vi "WinPositioner.vi"(0 "Display?":bool, 4 "Yoffset 2":dbl, 6 "Xoffset":dbl, 7 "Image":T1, 8 "Y position":dbl(slide) scale=0.0..10.0, 9 "Fine Y position":dbl(slide) scale=0.0..10.0, 10 "Fine X position":dbl(slide) scale=0.0..10.0, 11 "X position":dbl(slide) scale=0.0..10.0) -> (1 "Y position":dbl, 2 "X position":dbl, 5 "CGH_x":T1(plugin-control))   [LabVIEW 2011]
uses:
  <vilib>/vision/Image Controls.llb/IMAQ Image.ctl
panel:
  # "1"
  # "2"
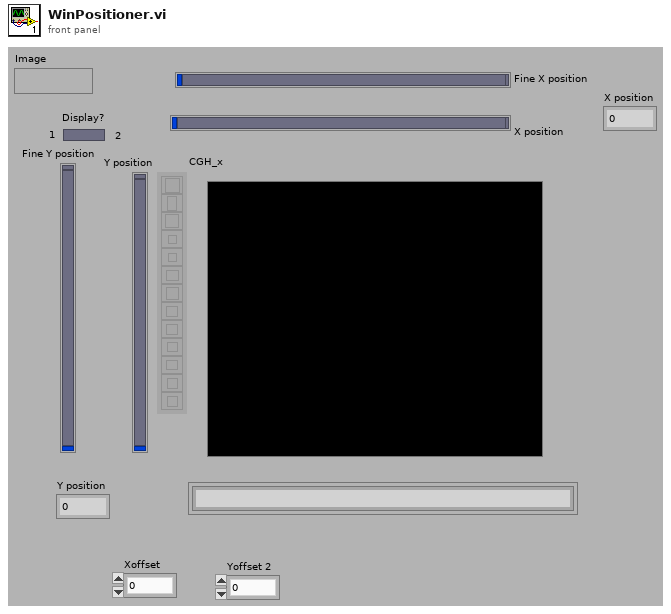
[diagram p1: front panel]
types:
  T1 = typedef "IMAQ Image.ctl" = refnum<image>
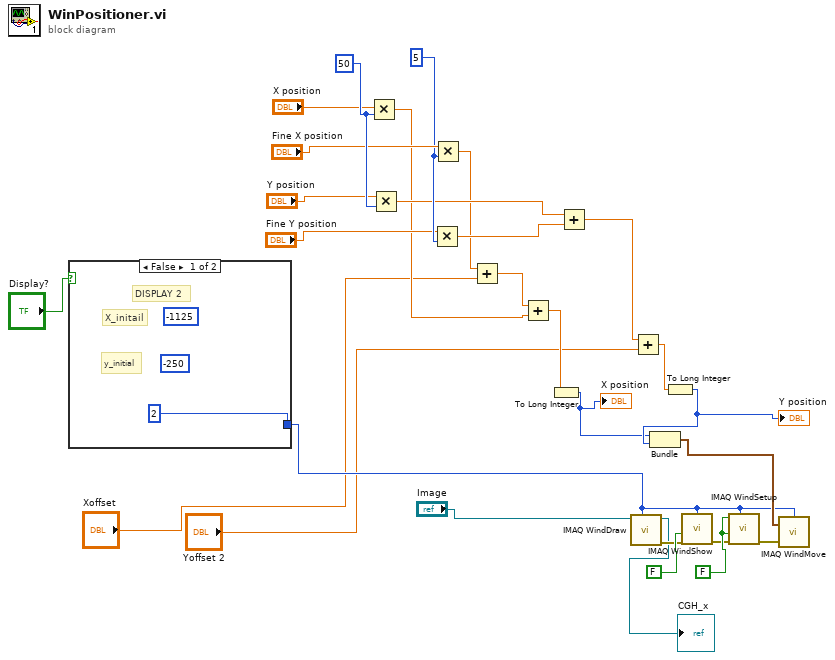
[diagram p0: block diagram]
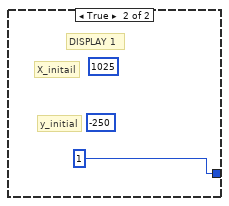
[diagram p2: hidden frame]
diagram:
  w18 = 5
  w21 = 50
  w27 = FALSE
  n1 = case shown="False" "Display?" {
    tunnel: [2 1] -> w5
    frame False {
      (unwired) -250
      (unwired) -1125
      # "DISPLAY 2"
      # "y_initial"
      # "X_initail"
    }
    frame True {
      (unwired) -250
      (unwired) 1025
      # "DISPLAY 1"
      # "y_initial"
      # "X_initail"
    }
  }
  n2 = Multiply(x="X position", y=w21) -> (x*y=w12:dbl)
  n3 = Multiply(x="Y position", y=w21) -> (x*y=w15:dbl)
  n4 = Multiply(x="Fine Y position", y=w18) -> (x*y=w14:dbl)
  n5 = Multiply(x="Fine X position", y=w18) -> (x*y=w13:dbl)
  n6 = Add(x=w13, y="Xoffset") -> (x+y=w11:dbl)
  n7 = Add(x=w11, y=w12) -> (x+y=w28:dbl)
  n8 = To Long Integer(number=w28) -> (32bit integer=w3:i32)
  "X position" <- w3
  n9 = Add(x=w15, y=w14) -> (x+y=w10:dbl)
  n10 = call "IMAQ WindDraw"("Window Number (0...15)"=w5, "Image"="Image") -> ("error out"=w23:errorcluster, "Image Out (duplicate)"=→"CGH_x":T1)  [unwired: 8 in]
  n11 = Add(x=w10, y="Yoffset 2") -> (x+y=w9:dbl)
  n12 = To Long Integer(number=w9) -> (32bit integer=w4:i32)
  "Y position" <- w4
  n13 = Bundle(w3, w4) -> (w6:cluster{i32, i32})  [unwired: 1 in]
  n14 = call "IMAQ WindShow"("error in (no error)"=w23, "Bring To Front? (N)"=FALSE, "Window Number (0...15)"=w5) -> ("error out"=w24:errorcluster)  [unwired: 3 in, 2 out]
  n15 = call "IMAQ WindSetup"("Window Number (0...15)"=w5, "error in (no error)"=w24, "Window has title bar? (Yes)"=w27, "Window can grow? (Yes)"=w27) -> ("error out"=w25:errorcluster)  [unwired: 7 in]
  n16 = call "IMAQ WindMove"("Window Number (0...15)"=w5, "Coordinates (screen)"=w6, "error in (no error)"=w25) -> ()  [unwired: 2 in, 2 out]
